vi "Unmarshal.vi"(8 "error in (no error)":errorcluster, 10 "Buffer":u8[](array[numeric]), 11 "int32 in":refnum<class "sint64.lvclass">) -> (0 "error out":errorcluster, 2 "Buffer Count":i32=8, 3 "int32 out":refnum<class "sint64.lvclass">)   [LabVIEW 2020, in "Protobuf RAW.lvlib" / "sint64.lvclass"]
uses:
  sint64.lvclass
  sint64.lvclass/sint64.ctl
  f4a157cf-4967-4c5b-a0d3-ce73e61944b8.vi
  f4a157cf-4967-4c5b-a0d3-ce73e61944b8.vi/e6afa5c7-117b-4965-af0c-e30c75561961.vi
  Protobuf RAW.lvlib
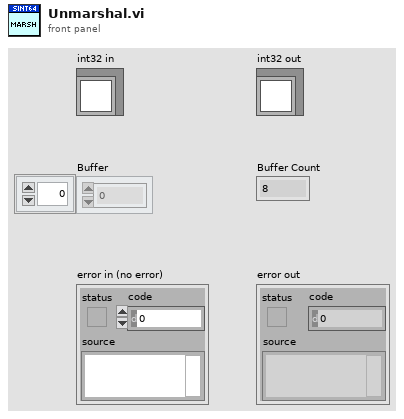
[diagram p1: front panel]
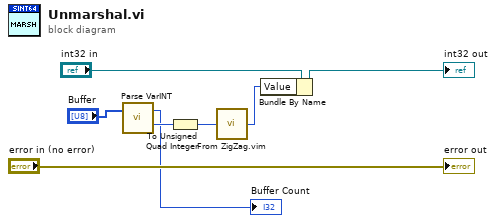
[diagram p0: block diagram]
diagram:
  n1 = call "Parse VarINT.vi"("Buffer"="Buffer") -> ("Numeric"=w4:u64, "Bytes"=→"Buffer Count":i32)  [unwired: 1 in]
  n2 = To Unsigned Quad Integer(1:w4) -> (0:w2:u64)
  n3 = call "From ZigZag.vim"("ZigZag"=w2) -> ("Signed Integer"=w3:i64)
  n4 = Bundle By Name(cluster="int32 in", "Value"=w3) -> (→"int32 out":refnum<class "sint64.lvclass">)
  "error out" <- "error in (no error)"
